vi "RealSense_HelloWorld_PointCloud Plus4.vi"() -> ()   [LabVIEW 2018]
doc: "Simple Demo showing how to connect a RealSense Camera to stream COLOR and DEPTH from the stereo camera of a D4xx series camera."
uses:
  <vilib>/Utility/miscctls.llb/LV3DPointTypeDef.ctl
  <vilib>/Utility/miscctls.llb/LVRGBAColorTypeDef.ctl
  libRealSense3.lvlib
  <vilib>/picture/3D Picture Control/NI_3D Picture Control.lvlib
panel:
  in  "Color format":enum16{"Monochrome", "RGB internal (RGB)"}(ring)
  in  "Display tab":T1(tab)
  out "depthUnits, um":i32=1000
  out "Stream selection":u16(ring)=5 items=["Depth + Left Color", "Unrectified L + R", "Rectified L + R", "Depth Only", "RGB ext. Only", "Depth + L Monochrome"]
  out "Found \nRealSense":bool=TRUE
  out "height, Y":i32=720
  out "width, X":i32=1280
  out "init results":T2={"camera name"="Intel RealSense D415", "camera S/N"="725112060262", "F/W"="05.09.11.00", "Sensor name"="Stereo Module", "api_version"=21100, "rscontext"=2785200371920, "device_list"=2783287753264, "device count"=2, "Dev out"=2783189103904, "sensor_list"=2783189110816, "sensor count"=2, "Sensor out"=2783184370480}
  in  "Select Resolution":u16(ring)=27 items=["424 x 240 @6fps", "424 x 240 @15fps", "424 x 240 @30fps", "424 x 240 @60fps", "424 x 240 @90fps", "480 x 270 @6fps", "480 x 270 @15fps", "480 x 270 @30fps", "480 x 270 @60fps", "480 x 270 @90fps", "640 x 360 @6fps", "640 x 360 @15fps", "640 x 360 @30fps", "640 x 360 @60fps", "640 x 360 @90fps", "640 x 480 @6fps", "640 x 480 @15fps", "640 x 480 @30fps", "640 x 480 @60fps", "640 x 480 @90fps", "848 x 100 @100fps", "848 x 480 @6fps", "848 x 480 @15fps", "848 x 480 @30fps", "848 x 480 @60fps", "848 x 480 @90fps", "1280 x 720 @6fps", "1280 x 720 @15fps", "1280 x 720 @30fps", "1280 x 800 @15fps", "1280 x 800 @30fps"]
  in  "Sensor index":i32
  in  "Device index":i32
  out "L-R Baseline, mm":sgl=55.142326
  out "fy":sgl=949.24713 format="%#_5g"
  out "fx":sgl=949.24713 format="%#_5g"
  out "ppy":sgl=364.42218 format="%#_5g"
  out "ppx":sgl=632.0836 format="%#_5g"
  out "Processed intrin out":T3={"width"=640, "height"=360, "ppx"=316.0418, "ppy"=182.21109, "fx"=474.62357, "fy"=474.62357, "model"=4, "coeffs[0]"=0.0, "coeffs[1]"=0.0, "coeffs[2]"=0.0, "coeffs[3]"=0.0, "coeffs[4]"=0.0} {"model" items=["RS_DISTORTION_NONE", "RS_DISTORTION_MODIFIED_BROWN_CONRADY", "RS_DISTORTION_INVERSE_BROWN_CONRADY", "RS_DISTORTION_FTHETA", "RS_DISTORTION_BROWN_CONRADY", "RS_DISTORTION_COUNT"]}
  in  "Exposure,us":sgl=33000.0
  in  "Autoexposure":bool=TRUE
  in  "Depth Presets":T4(ring)=enum."High Density"
  in  "Color Presets":T5(ring)=enum."DS410 (DS5a) 4"
  in  "Laser on/off":bool=TRUE
  in  "Gain(16-248)":sgl=16.0 min=16 max=248
  in  "Update Presets":bool
  in  "Laser \nPower (mW)":dbl(slide)=155.72448 min=0.0 max=360.0 scale=0.36..360.0
  in  "Range Scale":enum16{"200m", "100m", "60m", "6m", "2m", "1m"}(ring)=enum."6m"
  out "RGB image":picture
  out "Depth map":sgl[][](graph)
  in  "PostProcess":bool=TRUE
  out "Processing times":T6={"subsample, ms"=4, "depth-to-disp, ms"=1, "spatial filter, ms"=5, "temporal filter, ms"=1, "disp-to-depth, ms"=0}
  in  "Post-processing":T7={"Subsample"=TRUE, "Spatial filter"=TRUE, "Temporal filter"=TRUE}
  in  "Filter settings":T8={"Decimation Scale (1-10)"=3, "Spatial Alpha\n(0-1)"=0.6, "Spatial Delta \n(1/32 disp)"=8, "Temporal Alpha\n(0-1)"=0.4, "Temporal Delta\n(1/32 disp)"=20, "Persistence (0= none, 8=max)"=0, "spatial holefill radius\n(0 disable, 5 max) "=0, "spatial iteration\n(2=default)"=2} {"spatial iteration\n(2=default)" min=1 max=10; "Decimation Scale (1-10)" min=1 max=10; "Spatial Alpha\n(0-1)" min=0 max=1 format="%_2g"; "Spatial Delta \n(1/32 disp)" min=1; "Temporal Alpha\n(0-1)" min=0 max=1 format="%_2g"; "Temporal Delta\n(1/32 disp)" min=1; "Persistence (0= none, 8=max)" max=8; "spatial holefill radius\n(0 disable, 5 max)" max=6}
  out "3D Picture":refnum<vi>(3d-picture)
  in  "Texture":bool=TRUE
  out "Depth height":i32=360
  out "Depth width":i32=640
  out "Color Width":i32=1280
  out "Color Height":i32=720
  out "init error":string="No Error\rNo Error\rNo Error\rNo Error\rNo Error\rNo Error\rNo Error\rNo Error\rNo Error\rNo Error\rNo Error"
  out "Capture2 error":string="No Error"
  out "Start Error":string="No Error\rNo Error\rNo Error"
  out "Config error":string="No Error\rNo Error"
  out "Capture1 Error":string="No Error"
  out "Close Error":string="No Error\rNo Error\rNo Error\rNo Error"
  out "iteration":i32=29
  in  "stop":bool=TRUE
  # "RealSense Hello World: PointCloud & Post Processing"
  # "This demo shows how to connect a RealSense D4xx Stereo Depth Camera, and display the textured PointCloud."
  # "Note; When you change Depth Preset you need to stop and restart for the HDAD settings to take effect.\n\nTry the Color preset called \"Remove IR2\". It will remove the laser projector from the RGB 1280x720 image."
  # "INTRINSICS & EXTRINSICS"
  # "SELECT THE RESOLUTION"
  # "Recommendation:\nFor D435: 848x480, D415: 1280x720"
  # "DEPTH MAP"
  # "COLOR"
  # "Changes Color scale for Depth Map."
  # "20-1660000"
  # "3D POINTCLOUD"
  # "Rotate: Drag image\nMove X-Y: HOLD DOWN CTRL while dragging.\nZoom: SHIFT while dragging."
  # "ERRORS"
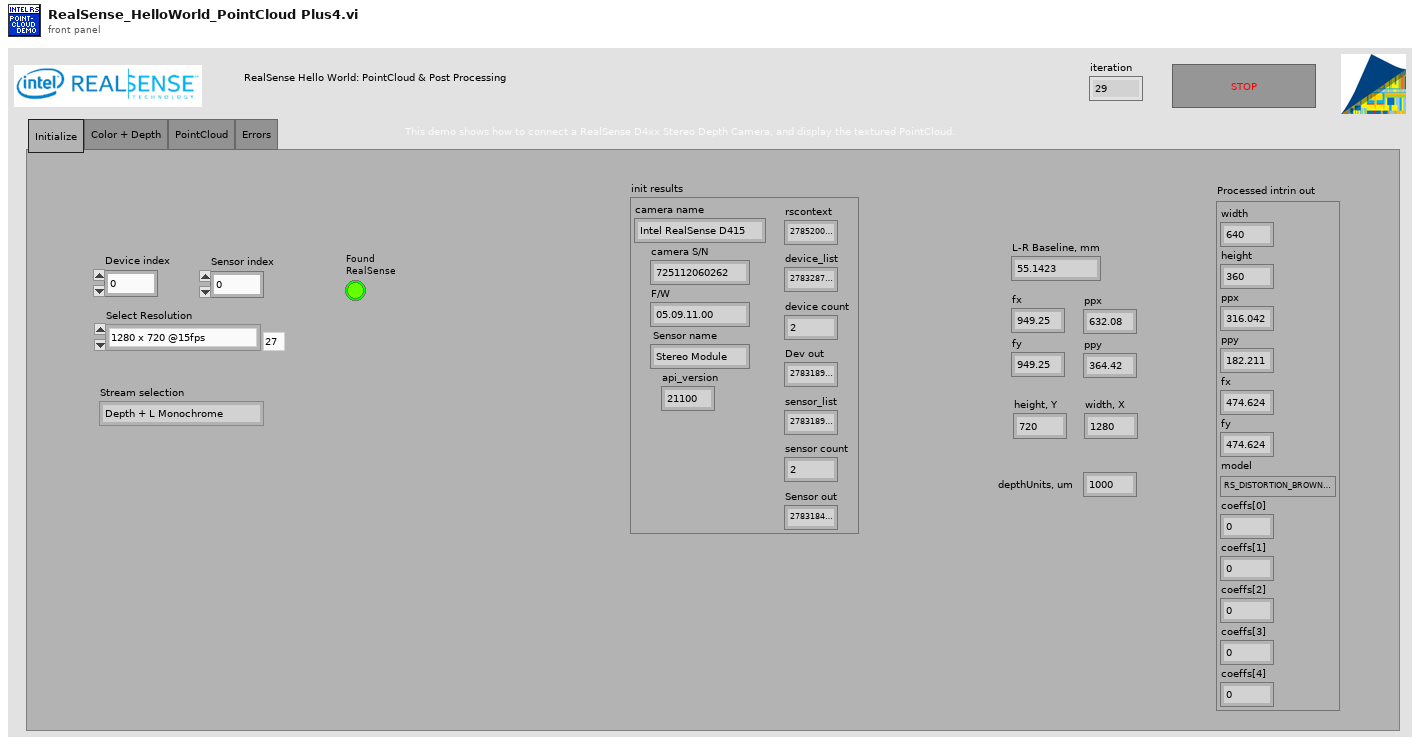
[diagram p1: front panel]
types:
  T1 = enum32{"Initialize", "Color + Depth", "PointCloud", "Errors"}
  T2 = cluster{"camera name":string, "camera S/N":string, "F/W":string, "Sensor name":string, "api_version":i32, "rscontext":u64, "device_list":u64, "device count":i32, "Dev out":u64, "sensor_list":u64, "sensor count":i32, "Sensor out":u64}
  T3 = cluster{"width":i32, "height":i32, "ppx":sgl, "ppy":sgl, "fx":sgl, "fy":sgl, "model":u32, "coeffs[0]":sgl, "coeffs[1]":sgl, "coeffs[2]":sgl, "coeffs[3]":sgl, "coeffs[4]":sgl}
  T4 = enum16{"Custom", "Original", "New Depth 1", "New Depth 2", "Depth Active 1", "Active 3D Scan", "Active Short A", "Active Short C", "Face", "Face2", "Best Box", "High Density", "Medium Density", "High Accuracy", "Hand", "Short Range", "Flat wall", "Load .JSON", "Load .JSON2"}
  T5 = enum16{"Custom", "RS400 (DS5p)", "RS400 (DS5p) 2", "RS400 (DS5p) 3", "RS400 (DS5p) 4", "RS400 (DS5p) 5", "RS410 (DS5a)", "RS410 (DS5a) 2", "DS410 (DS5a) 3", "DS410 (DS5a) 4", "DS410+IR", "DS5LR", "DS5LR-2", "DS5LR no pattern", "RS410 Remove IR", "RS410 Remove IR 2", "DS5micro", "D435"}
  T6 = cluster{"subsample, ms":u32, "depth-to-disp, ms":u32, "spatial filter, ms":u32, "temporal filter, ms":u32, "disp-to-depth, ms":u32}
  T7 = cluster{"Subsample":bool, "Spatial filter":bool, "Temporal filter":bool}
  T8 = cluster{"Decimation Scale (1-10)":u8, "Spatial Alpha\n(0-1)":sgl, "Spatial Delta \n(1/32 disp)":u16, "Temporal Alpha\n(0-1)":sgl, "Temporal Delta\n(1/32 disp)":u16, "Persistence (0= none, 8=max)":u8, "spatial holefill radius\n(0 disable, 5 max) ":u8, "spatial iteration\n(2=default)":u8}
  T9 = cluster{"Decimation Scale (1-10)":u8, "Spatial Alpha\n(0-1)":sgl, "Spatial Delta \n(1/32 disp)":u16, "Temporal Alpha\n(0-1)":sgl, "Temporal Delta\n(1/32 disp)":u16, "Persistence (0= none, 8=max)":u8, "spatial holefill radius\n(0 disable, 6 max) ":u8, "spatial iteration\n(2=default)":u8}
  T10 = cluster{"width":i32, "height":i32, "fps":i32, "Profile":u64, "ppx":sgl, "ppy":sgl, "fx":sgl, "fy":sgl, "model":u32}
  T11 = cluster{"decimation filter queue":u64, "spatial filter queue":u64, "temporal filter queue":u64, "disparity_transforg_2_queue":u64, "disparity_transforg_1_queue":u64}
  T12 = cluster{"decimation filter block":u64, "spatial filter block":u64, "temporal filter block":u64, "disparity_transforg_2_block":u64, "disparity_transforg_1_block":u64}
  T13 = enum16{"Points", "Lines", "Line Strip", "Line Loop", "Triangles", "Triangle Strip", "Triangle Fan", "Quads", "Quad Strip", "Polygon"}
  T14 = typedef "LVRGBAColorTypeDef.ctl" = cluster{"Red":sgl, "Green":sgl, "Blue":sgl, "Alpha":sgl}
  T15 = enum16{"Overall", "Per Primitive", "Per Vertex", "Binding Off"}
  T16 = cluster{"Decimation Scale (1-10)":bool, "Spatial Alpha\n(0-1)":bool, "Spatial Delta \n(1/32 disp)":bool, "Temporal Alpha\n(0-1)":bool, "Temporal Delta\n(1/32 disp)":bool, "Persistence (0= none, 8=max)":bool, bool, "spatial iteration\n(2=default)":bool}
  T17 = enum16{"Depth", "Color (ext.)", "Color (left) ", "IR Left", "IR Right", "IR Left (Y16)", "IR Right (Y16)"}
  T18 = cluster{"R":dbl, "G":dbl, "B":dbl, "Alpha":dbl}[]
  T19 = typedef "LV3DPointTypeDef.ctl" = cluster{"X":sgl, "Y":sgl, "Z":sgl}
  T20 = cluster{"Alpha":sgl, "Blue":sgl, "Green":sgl, "Red":sgl}
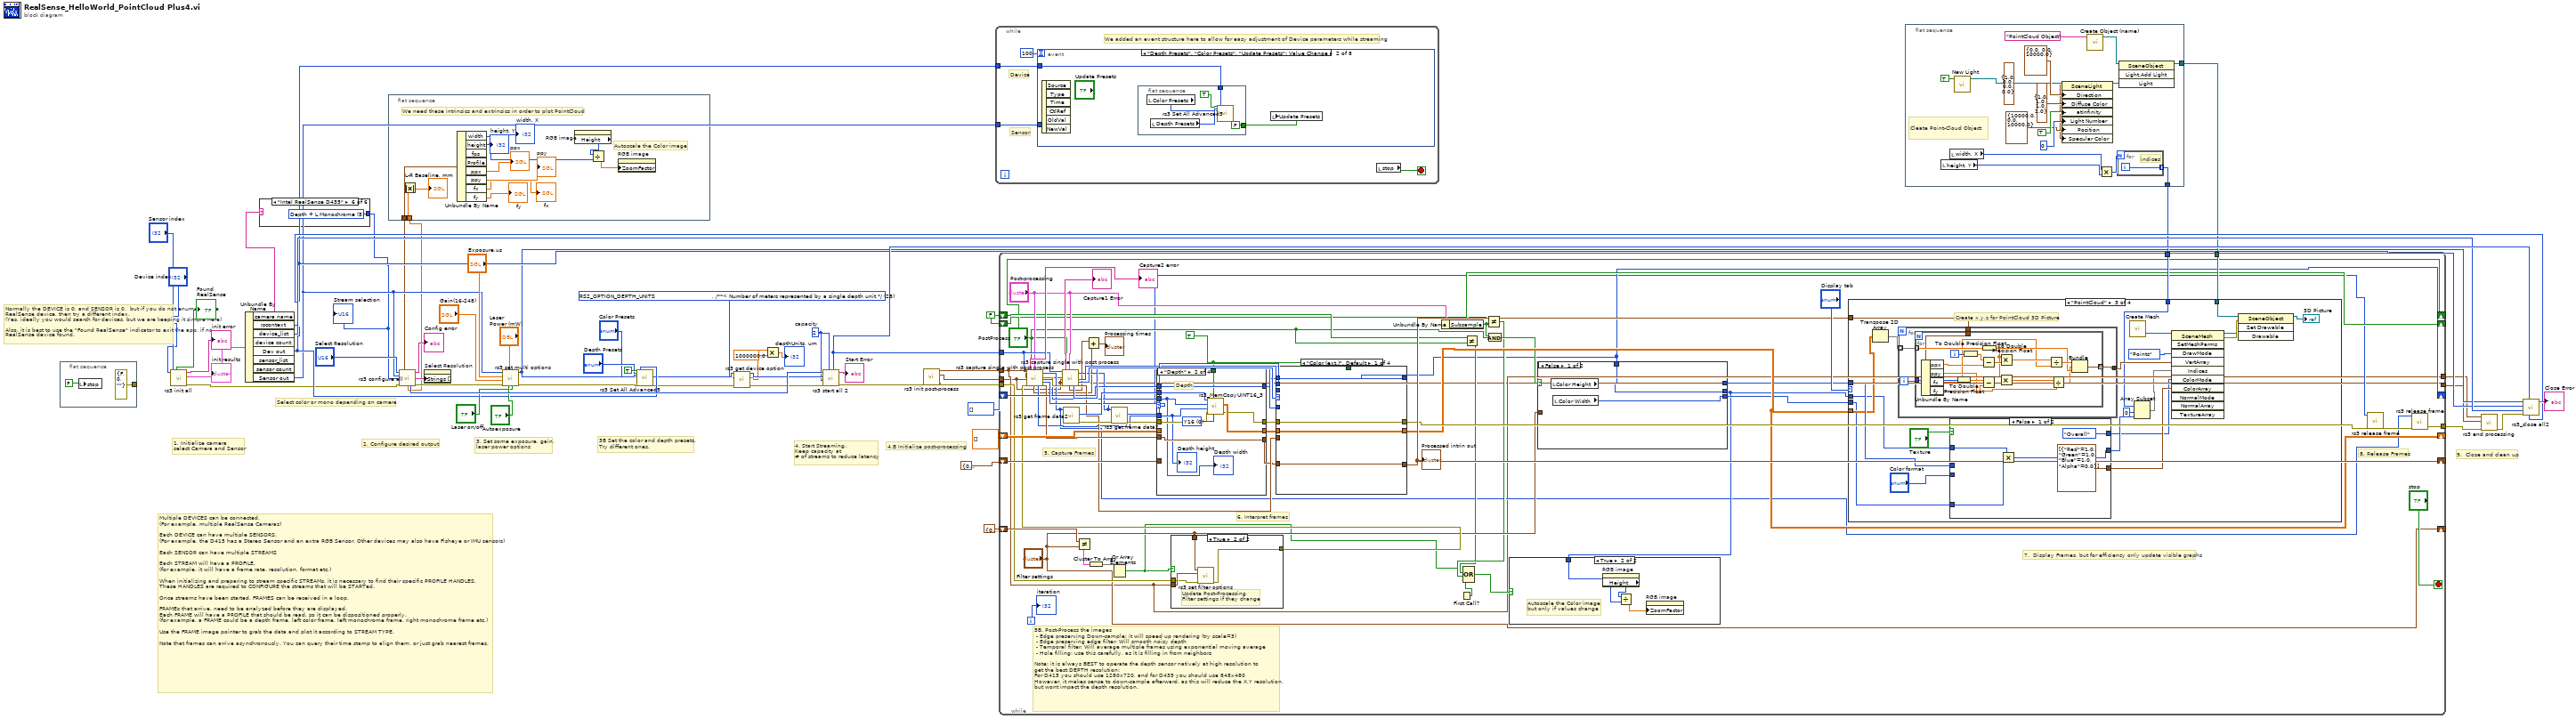
[diagram p0: block diagram]
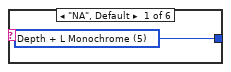
[diagram p2: hidden frame]
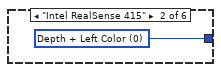
[diagram p3: hidden frame]
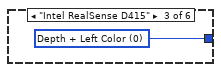
[diagram p4: hidden frame]
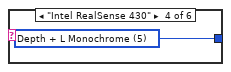
[diagram p5: hidden frame]
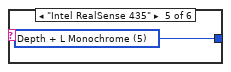
[diagram p6: hidden frame]
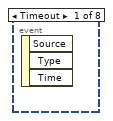
[diagram p7: hidden frame]
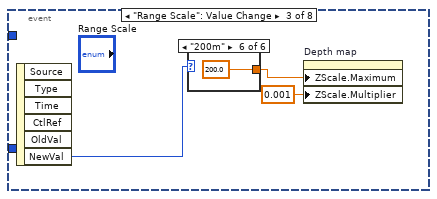
[diagram p8: hidden frame]
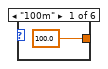
[diagram p9: hidden frame]
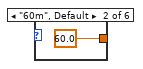
[diagram p10: hidden frame]
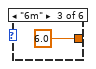
[diagram p11: hidden frame]
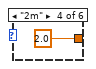
[diagram p12: hidden frame]
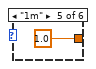
[diagram p13: hidden frame]
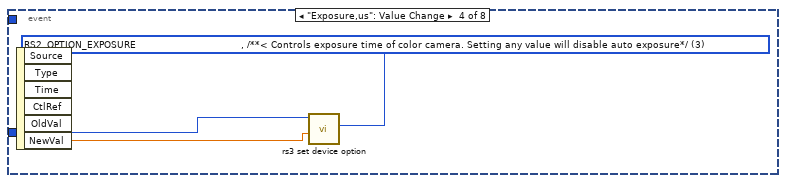
[diagram p14: hidden frame]
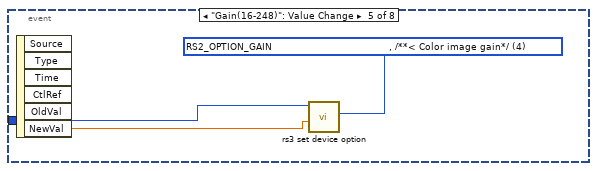
[diagram p15: hidden frame]
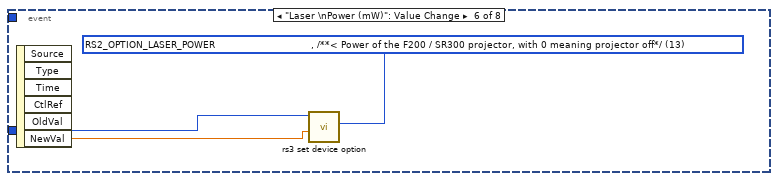
[diagram p16: hidden frame]
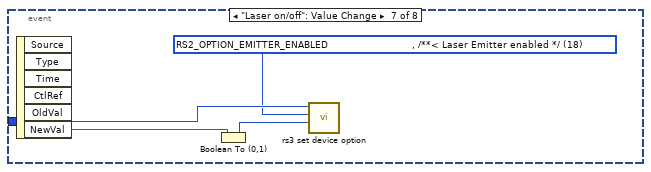
[diagram p17: hidden frame]
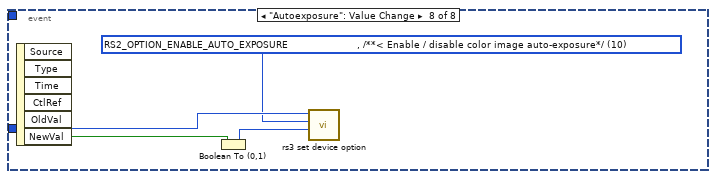
[diagram p18: hidden frame]
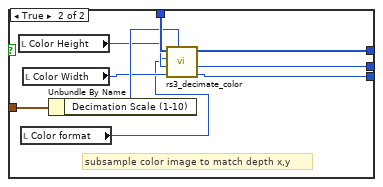
[diagram p20: hidden frame]
diagram:
  w6 = FALSE ("PostProcess")
  w13 = 2  # capacity
  w17 = u16 28 items=["    RS2_OPTION_BACKLIGHT_COMPENSATION                     , /**< Enable / disable color backlight compensation*/", "    RS2_OPTION_BRIGHTNESS                                 , /**< Color image brightness*/", "    RS2_OPTION_CONTRAST                                   , /**< Color image contrast*/", "    RS2_OPTION_EXPOSURE                                   , /**< Controls exposure time of color camera. Setting any value will disable auto exposure*/", "    RS2_OPTION_GAIN                                       , /**< Color image gain*/", "    RS2_OPTION_GAMMA                                      , /**< Color image gamma setting*/", "    RS2_OPTION_HUE                                        , /**< Color image hue*/", "    RS2_OPTION_SATURATION                                 , /**< Color image saturation setting*/", "    RS2_OPTION_SHARPNESS                                  , /**< Color image sharpness setting*/", "    RS2_OPTION_WHITE_BALANCE                              , /**< Controls white balance of color image. Setting any value will disable auto white balance*/", "    RS2_OPTION_ENABLE_AUTO_EXPOSURE                       , /**< Enable / disable color image auto-exposure*/", "    RS2_OPTION_ENABLE_AUTO_WHITE_BALANCE                  , /**< Enable / disable color image auto-white-balance*/", "    RS2_OPTION_VISUAL_PRESET                              , /**< Provide access to several recommend sets of option presets for the depth camera */", "    RS2_OPTION_LASER_POWER                                , /**< Power of the F200 / SR300 projector, with 0 meaning projector off*/", "    RS2_OPTION_ACCURACY                                   , /**< Set the number of patterns projected per frame. The higher the accuracy value the more patterns projected. Increasing the number of patterns help to achieve better accuracy. Note that this c", "    RS2_OPTION_MOTION_RANGE                               , /**< Motion vs. Range trade-off, with lower values allowing for better motion sensitivity and higher values allowing for better depth range*/", "    RS2_OPTION_FILTER_OPTION                              , /**< Set the filter to apply to each depth frame. Each one of the filter is optimized per the application requirements*/", "    RS2_OPTION_CONFIDENCE_THRESHOLD                       , /**< The confidence level threshold used by the Depth algorithm pipe to set whether a pixel will get a valid range or will be marked with invalid range*/", "    RS2_OPTION_EMITTER_ENABLED                            , /**< Laser Emitter enabled */", "    RS2_OPTION_FRAMES_QUEUE_SIZE                          , /**< Number of frames the user is allowed to keep per stream. Trying to hold-on to more frames will cause frame-drops.*/", "    RS2_OPTION_TOTAL_FRAME_DROPS                          , /**< Total number of detected frame drops from all streams */", "    RS2_OPTION_AUTO_EXPOSURE_MODE                         , /**< Auto-Exposure modes: Static, Anti-Flicker and Hybrid */", "    RS2_OPTION_POWER_LINE_FREQUENCY                       , /**< Power Line Frequency control for anti-flickering Off/50Hz/60Hz/Auto */", "    RS2_OPTION_ASIC_TEMPERATURE                           , /**< Current Asic Temperature */", "    RS2_OPTION_ERROR_POLLING_ENABLED                      , /**< disable error handling */", "    RS2_OPTION_PROJECTOR_TEMPERATURE                      , /**< Current Projector Temperature */", "    RS2_OPTION_OUTPUT_TRIGGER_ENABLED                     , /**< Enable / disable trigger to be outputed from the camera to any external device on every depth frame */", "    RS2_OPTION_MOTION_MODULE_TEMPERATURE                  , /**< Current Motion-Module Temperature */", "    RS2_OPTION_DEPTH_UNITS                                , /**< Number of meters represented by a single depth unit */", "    RS2_OPTION_ENABLE_MOTION_CORRECTION                   , /**< Enable/Disable automatic correction of the motion data */", "    RS2_OPTION_AUTO_EXPOSURE_PRIORITY                     , /**< Allows sensor to dynamically ajust the frame rate depending on lighting conditions */", "    RS2_OPTION_COLOR_SCHEME                               , /**< Color scheme for data visualization */", "    RS2_OPTION_HISTOGRAM_EQUALIZATION_ENABLED             , /**< Perform histogram equalization post-processing on the depth data */", "    RS2_OPTION_MIN_DISTANCE                               , /**< Minimal distance to the target */", "    RS2_OPTION_MAX_DISTANCE                               , /**< Maximum distance to the target */", "    RS2_OPTION_TEXTURE_SOURCE                             , /**< Texture mapping stream unique ID */", "    RS2_OPTION_FILTER_MAGNITUDE                           , /**< The 2D-filter effect. The specific interpretation is given within the context of the filter */", "    RS2_OPTION_FILTER_SMOOTH_ALPHA                        , /**< 2D-filter parameter controls the weight/radius for smoothing.*/", "    RS2_OPTION_FILTER_SMOOTH_DELTA                        , /**< 2D-filter range/validity threshold*/", "    RS2_OPTION_HOLES_FILL                                 , /**< Enhance depth data post-processing with holes filling where appropriate*/", "    RS2_OPTION_STEREO_BASELINE                            , /**< The distance in mm between the first and the second imagers in stereo-based depth cameras*/", "    RS2_OPTION_AUTO_EXPOSURE_CONVERGE_STEP                , /**< Allows dynamically ajust the converge step value of the target exposure in Auto-Exposure algorithm*/", "    RS2_OPTION_COUNT                                        /**< Number of enumeration values. Not a valid input: intended to be used in for-loops. */"] ("RS Option")
  # "4.B Initialize post-processing"
  # "4. Start Streaming. \nKeep capacity at \n# of streams to reduce latency"
  # "3B Set the color and depth presets.\nTry different ones."
  # "Select color or mono depending on camera"
  # "Normally the DEVICE is 0, and SENSOR is 0,  but if you do not enumerate the RealSense device, then try a different index.\n(Yes, ideally you would search for devices, but we are keeping it simple here)\n\nAlso, it is best to use the \"Found RealSense\" indicator to exit the app, if no RealSense device found."
  # "Multiple DEVICES can be connected. \n(For example, multiple RealSense Cameras)\n\nEach DEVICE can have multiple SENSORS. \n(For example, the D415 has a Stereo Sensor and an extra RGB Sensor. Other devices may also have Fisheye or IMU sensors) \n\nEach SENSOR can have multiple STREAMS\n\nEach STREAM will have a PROFILE. \n(for example, it will have a frame rate, resolution, format etc.)\n\nWhen initializing and preparing to stream specific STREAMs, it is necessary to find their specific PROFILE HANDLES.\nThese HANDLES are required to CONFIGURE the streams that will be STARTed. \n\nOnce streams have been started, FRAMES can be received in a loop. \n \nFRAMEs that arrive, need to be analyzed before they are displayed. \nEach FRAME will have a PROFILE that should be read, so it can be dispositioned properly.\n(for example, a FRAME could be a depth frame, left color frame, left monochrome frame, right monochrome frame etc.)\n\nUse the FRAME image pointer to grab the data and plot it according to STREAM TYPE.\n\nNote that frames can arrive asynchronously. You can query their time stamp to align them, or just grab nearest frames."
  # "9.  Close and clean up"
  # "3. Set some exposure, gain, \nlaser power options"
  # "2. Configure desired output"
  # "1. Initialize camera\nselect Camera and Sensor"
  n1 = flat-sequence {
    tunnel: [errorcluster {"status"=FALSE, "code"=0, "source"=""} ("error in")] -> _
    frame #0 {
      n2 = local write "stop"(FALSE ("stop")) -> ()
    }
  }
  n3 = call "rs3 init all.vi"("Select Device"="Device index", "Select Sensor"="Sensor index") -> ("error out"=w23:errorcluster, "init results"=w28:T2, "init error"=→"init error":string, "Found RealSense"=→"Found \nRealSense":bool)  [unwired: 3 in, 3 out]
  "init results" <- w28
  n4 = Unbundle By Name(w28) -> ("camera name"=w22:string, "rscontext"=w50:u64, "device_list"=w51:u64, "Dev out"=w36:u64, "Sensor out"=w35:u64)  [unwired: 3 out]
  n5 = case shown="\"Intel RealSense D435\"" w22 {
    tunnel: [w58 w59 w60 w61 w62 w63] -> w5
    frame "NA", Default {
      w58 = u16 5 items=["Depth + Left Color", "Unrectified L + R", "Rectified L + R", "Depth Only", "RGB ext. Only", "Depth + L Monochrome"] ("Stream selection")
    }
    frame "Intel RealSense 415" {
      w59 = u16 0 items=["Depth + Left Color", "Unrectified L + R", "Rectified L + R", "Depth Only", "RGB ext. Only", "Depth + L Monochrome"] ("Stream selection")
    }
    frame "Intel RealSense D415" {
      w60 = u16 0 items=["Depth + Left Color", "Unrectified L + R", "Rectified L + R", "Depth Only", "RGB ext. Only", "Depth + L Monochrome"] ("Stream selection")
    }
    frame "Intel RealSense 430" {
      w61 = u16 5 items=["Depth + Left Color", "Unrectified L + R", "Rectified L + R", "Depth Only", "RGB ext. Only", "Depth + L Monochrome"] ("Stream selection")
    }
    frame "Intel RealSense 435" {
      w62 = u16 5 items=["Depth + Left Color", "Unrectified L + R", "Rectified L + R", "Depth Only", "RGB ext. Only", "Depth + L Monochrome"] ("Stream selection")
    }
    frame "Intel RealSense D435" {
      w63 = u16 5 items=["Depth + Left Color", "Unrectified L + R", "Rectified L + R", "Depth Only", "RGB ext. Only", "Depth + L Monochrome"] ("Stream selection")
    }
  }
  "Stream selection" <- w5
  n6 = flat-sequence {
    tunnel: w33 -> [w74]
    tunnel: w32 -> [w73]
    frame #0 {
      # "Autoscale the Color image"
      # "We need these intrinsics and extrinsics in order to plot PointCloud"
      n7 = Absolute Value(x=w74) -> (abs(x)=→"L-R Baseline, mm":sgl)
      n8 = Unbundle By Name(w73) -> ("width"=→"width, X":i32, "height"=w71:i32, "ppx"=→"ppx":sgl, "ppy"=→"ppy":sgl, "fx"=→"fx":sgl, "fy"=→"fy":sgl)  [unwired: 2 out]
      "height, Y" <- w71
      n9 = property on="RGB image" class="Pict"() -> ("Height"=w72:u32)  [unwired: 2 in, 2 out]
      n10 = Divide(x=w72, y=w71) -> (x/y=w70:dbl)
      n11 = property on="RGB image" class="Pict"("ZoomFactor"=w70) -> ()  [unwired: 2 in, 2 out]
    }
  }
  n12 = call "rs3 configure all.vi"("Select Resolution"="Select Resolution", "Sensor in"=w35, "Stream selection"=w5, "error in (no error)"=w23) -> ("Output stream L"=w32:T10, "config error"=→"Config error":string, "Output stream"=w47:string[], "L-R Baseline, mm"=w33:sgl, "Stream Profile Handles"=w55:u64[], "error out"=w46:errorcluster)  [unwired: 2 in, 4 out]
  n13 = property on="Select Resolution" class="Ring (strict)"("Strings []"=w47) -> ()  [unwired: 2 in, 2 out]
  n14 = call "rs3 set multi options.vi"("laser on/off"="Laser on/off", "autoexposure"="Autoexposure", "Laser power, mW (0-360)"="Laser \nPower (mW)", "error in (no error)"=w46, "Gain(16-248)"="Gain(16-248)", "Exposure, us"="Exposure,us", "Sensor in"=w35) -> ("error out"=w40:errorcluster, "Sensor out"=w19:u64)  [unwired: 2 in, 1 out]
  n15 = call "rs3 Set All Advanced5.vi"("Set Color Corr"=TRUE, "Depth Presets"="Depth Presets", "Color Presets"="Color Presets", "error in (no error)"=w40, "device in"=w36) -> ("error out"=w21:errorcluster)  [unwired: 20 in, 2 out]
  n16 = call "rs3 get device option.vi"("error in (no error)"=w21, "RS Option"=w17, "sensor in"=w19) -> ("error out"=w20:errorcluster, "option return"=w16:dbl, "sensor out"=w18:u64)  [unwired: 4 in, 2 out]
  n17 = Multiply(x=w16, y=1000000.0) -> (x*y=→"depthUnits, um":dbl)
  n18 = call "rs3 start all 2.vi"("capacity"=w13, "error in (no error)"=w20, "Count of Streams"=w13, "Sensor in"=w18, "Stream profile array"=w55) -> ("error out"=w12:errorcluster, "Config Error"=→"Start Error":string, "queue out"=w54:u64)  [unwired: 3 in, 1 out]
  n19 = call "rs3 init post-process.vi"("error in (no error)"=w12) -> ("error out"=w7:errorcluster, "Processing Queues"=w11:T11, "Processing Blocks"=w10:T12)  [unwired: 8 in]
  n20 = while {
    tunnel: w36 -> [w77]
    tunnel: w35 -> [w76]
    stop <- w78 stop-if-true
    # "Sensor"
    # "Device"
    # "We added an event structure here to allow for easy adjustment of Device parameters while streaming"
    n21 = event shown="[1] \"Depth Presets\", \"Color Presets\", \"Update Presets\": Value Change" {
      selector: _ -> [_ _ _ _ _ _ _ _]
      dyn-events: _ -> [_ _ _ _ _ _ _ _]
      timeout: 100 -> [_ _ _ _ _ _ _ _]
      tunnel: w77 -> [_ w80 _ _ _ _ _ _]
      tunnel: w76 -> [_ _ _ w97 w100 w103 w107 w111]
      event Timeout {
        n22 = event-data() -> ()  [unwired: 1 in, 3 out]
      }
      event "Depth Presets", "Color Presets", "Update Presets": Value Change {
        n23 = event-data() -> ()  [unwired: 1 in, 6 out]
        n24 = flat-sequence {
          tunnel: w80 -> [w82]
          tunnel: [FALSE ("Update Presets")] -> w79
          frame #0 {
            n25 = local read "Color Presets"() -> (w84:T5)
            n26 = local read "Depth Presets"() -> (w85:T4)
            n27 = call "rs3 Set All Advanced5.vi"("Set Color Corr"=TRUE, "Depth Presets"=w85, "Color Presets"=w84, "device in"=w82) -> ()  [unwired: 21 in, 3 out]
          }
        }
        n28 = local write "Update Presets"(w79) -> ()
      }
      event "Range Scale": Value Change {
        n29 = event-data() -> ("NewVal"=w87:enum16{"200m", "100m", "60m", "6m", "2m", "1m"})  [unwired: 1 in, 5 out]
        n30 = case shown="\"200m\"" w87 {
          tunnel: [100.0 ("Z Scale.Offset and Multiplier:Multiplier") 60.0 ("Z Scale.Offset and Multiplier:Multiplier") 6.0 ("Z Scale.Offset and Multiplier:Multiplier") 2.0 ("Z Scale.Offset and Multiplier:Multiplier") 1.0 ("Z Scale.Offset and Multiplier:Multiplier") 200.0 ("Z Scale.Offset and Multiplier:Multiplier")] -> w86
          frame "100m" {
          }
          frame "60m", Default {
          }
          frame "6m" {
          }
          frame "2m" {
          }
          frame "1m" {
          }
          frame "200m" {
          }
        }
        n31 = property on="Depth map" class="IntGraph (strict)"("ZScale.Maximum"=w86, "ZScale.Multiplier"=0.001 ("Z Scale.Offset and Multiplier:Multiplier")) -> ()  [unwired: 2 in, 2 out]
      }
      event "Exposure,us": Value Change {
        w95 = u16 3 items=["    RS2_OPTION_BACKLIGHT_COMPENSATION                     , /**< Enable / disable color backlight compensation*/", "    RS2_OPTION_BRIGHTNESS                                 , /**< Color image brightness*/", "    RS2_OPTION_CONTRAST                                   , /**< Color image contrast*/", "    RS2_OPTION_EXPOSURE                                   , /**< Controls exposure time of color camera. Setting any value will disable auto exposure*/", "    RS2_OPTION_GAIN                                       , /**< Color image gain*/", "    RS2_OPTION_GAMMA                                      , /**< Color image gamma setting*/", "    RS2_OPTION_HUE                                        , /**< Color image hue*/", "    RS2_OPTION_SATURATION                                 , /**< Color image saturation setting*/", "    RS2_OPTION_SHARPNESS                                  , /**< Color image sharpness setting*/", "    RS2_OPTION_WHITE_BALANCE                              , /**< Controls white balance of color image. Setting any value will disable auto white balance*/", "    RS2_OPTION_ENABLE_AUTO_EXPOSURE                       , /**< Enable / disable color image auto-exposure*/", "    RS2_OPTION_ENABLE_AUTO_WHITE_BALANCE                  , /**< Enable / disable color image auto-white-balance*/", "    RS2_OPTION_VISUAL_PRESET                              , /**< Provide access to several recommend sets of option presets for the depth camera */", "    RS2_OPTION_LASER_POWER                                , /**< Power of the F200 / SR300 projector, with 0 meaning projector off*/", "    RS2_OPTION_ACCURACY                                   , /**< Set the number of patterns projected per frame. The higher the accuracy value the more patterns projected. Increasing the number of patterns help to achieve better accuracy. Note that this c", "    RS2_OPTION_MOTION_RANGE                               , /**< Motion vs. Range trade-off, with lower values allowing for better motion sensitivity and higher values allowing for better depth range*/", "    RS2_OPTION_FILTER_OPTION                              , /**< Set the filter to apply to each depth frame. Each one of the filter is optimized per the application requirements*/", "    RS2_OPTION_CONFIDENCE_THRESHOLD                       , /**< The confidence level threshold used by the Depth algorithm pipe to set whether a pixel will get a valid range or will be marked with invalid range*/", "    RS2_OPTION_EMITTER_ENABLED                            , /**< Laser Emitter enabled */", "    RS2_OPTION_FRAMES_QUEUE_SIZE                          , /**< Number of frames the user is allowed to keep per stream. Trying to hold-on to more frames will cause frame-drops.*/", "    RS2_OPTION_TOTAL_FRAME_DROPS                          , /**< Total number of detected frame drops from all streams */", "    RS2_OPTION_AUTO_EXPOSURE_MODE                         , /**< Auto-Exposure modes: Static, Anti-Flicker and Hybrid */", "    RS2_OPTION_POWER_LINE_FREQUENCY                       , /**< Power Line Frequency control for anti-flickering Off/50Hz/60Hz/Auto */", "    RS2_OPTION_ASIC_TEMPERATURE                           , /**< Current Asic Temperature */", "    RS2_OPTION_ERROR_POLLING_ENABLED                      , /**< disable error handling */", "    RS2_OPTION_PROJECTOR_TEMPERATURE                      , /**< Current Projector Temperature */", "    RS2_OPTION_OUTPUT_TRIGGER_ENABLED                     , /**< Enable / disable trigger to be outputed from the camera to any external device on every depth frame */", "    RS2_OPTION_MOTION_MODULE_TEMPERATURE                  , /**< Current Motion-Module Temperature */", "    RS2_OPTION_DEPTH_UNITS                                , /**< Number of meters represented by a single depth unit */", "    RS2_OPTION_ENABLE_MOTION_CORRECTION                   , /**< Enable/Disable automatic correction of the motion data */", "    RS2_OPTION_AUTO_EXPOSURE_PRIORITY                     , /**< Allows sensor to dynamically ajust the frame rate depending on lighting conditions */", "    RS2_OPTION_COUNT                                      , /**< Number of enumeration values. Not a valid input: intended to be used in for-loops. */"] ("RS Option")
        n32 = event-data() -> ("NewVal"=w96:sgl)  [unwired: 1 in, 5 out]
        n33 = call "rs3 set device option.vi"("value"=w96, "RS Option"=w95, "Sensor in"=w97) -> ()  [unwired: 6 in, 3 out]
      }
      event "Gain(16-248)": Value Change {
        w98 = u16 4 items=["    RS2_OPTION_BACKLIGHT_COMPENSATION                     , /**< Enable / disable color backlight compensation*/", "    RS2_OPTION_BRIGHTNESS                                 , /**< Color image brightness*/", "    RS2_OPTION_CONTRAST                                   , /**< Color image contrast*/", "    RS2_OPTION_EXPOSURE                                   , /**< Controls exposure time of color camera. Setting any value will disable auto exposure*/", "    RS2_OPTION_GAIN                                       , /**< Color image gain*/", "    RS2_OPTION_GAMMA                                      , /**< Color image gamma setting*/", "    RS2_OPTION_HUE                                        , /**< Color image hue*/", "    RS2_OPTION_SATURATION                                 , /**< Color image saturation setting*/", "    RS2_OPTION_SHARPNESS                                  , /**< Color image sharpness setting*/", "    RS2_OPTION_WHITE_BALANCE                              , /**< Controls white balance of color image. Setting any value will disable auto white balance*/", "    RS2_OPTION_ENABLE_AUTO_EXPOSURE                       , /**< Enable / disable color image auto-exposure*/", "    RS2_OPTION_ENABLE_AUTO_WHITE_BALANCE                  , /**< Enable / disable color image auto-white-balance*/", "    RS2_OPTION_VISUAL_PRESET                              , /**< Provide access to several recommend sets of option presets for the depth camera */", "    RS2_OPTION_LASER_POWER                                , /**< Power of the F200 / SR300 projector, with 0 meaning projector off*/", "    RS2_OPTION_ACCURACY                                   , /**< Set the number of patterns projected per frame. The higher the accuracy value the more patterns projected. Increasing the number of patterns help to achieve better accuracy. Note that this c", "    RS2_OPTION_MOTION_RANGE                               , /**< Motion vs. Range trade-off, with lower values allowing for better motion sensitivity and higher values allowing for better depth range*/", "    RS2_OPTION_FILTER_OPTION                              , /**< Set the filter to apply to each depth frame. Each one of the filter is optimized per the application requirements*/", "    RS2_OPTION_CONFIDENCE_THRESHOLD                       , /**< The confidence level threshold used by the Depth algorithm pipe to set whether a pixel will get a valid range or will be marked with invalid range*/", "    RS2_OPTION_EMITTER_ENABLED                            , /**< Laser Emitter enabled */", "    RS2_OPTION_FRAMES_QUEUE_SIZE                          , /**< Number of frames the user is allowed to keep per stream. Trying to hold-on to more frames will cause frame-drops.*/", "    RS2_OPTION_TOTAL_FRAME_DROPS                          , /**< Total number of detected frame drops from all streams */", "    RS2_OPTION_AUTO_EXPOSURE_MODE                         , /**< Auto-Exposure modes: Static, Anti-Flicker and Hybrid */", "    RS2_OPTION_POWER_LINE_FREQUENCY                       , /**< Power Line Frequency control for anti-flickering Off/50Hz/60Hz/Auto */", "    RS2_OPTION_ASIC_TEMPERATURE                           , /**< Current Asic Temperature */", "    RS2_OPTION_ERROR_POLLING_ENABLED                      , /**< disable error handling */", "    RS2_OPTION_PROJECTOR_TEMPERATURE                      , /**< Current Projector Temperature */", "    RS2_OPTION_OUTPUT_TRIGGER_ENABLED                     , /**< Enable / disable trigger to be outputed from the camera to any external device on every depth frame */", "    RS2_OPTION_MOTION_MODULE_TEMPERATURE                  , /**< Current Motion-Module Temperature */", "    RS2_OPTION_DEPTH_UNITS                                , /**< Number of meters represented by a single depth unit */", "    RS2_OPTION_ENABLE_MOTION_CORRECTION                   , /**< Enable/Disable automatic correction of the motion data */", "    RS2_OPTION_AUTO_EXPOSURE_PRIORITY                     , /**< Allows sensor to dynamically ajust the frame rate depending on lighting conditions */", "    RS2_OPTION_COUNT                                      , /**< Number of enumeration values. Not a valid input: intended to be used in for-loops. */"] ("RS Option")
        n34 = event-data() -> ("NewVal"=w99:sgl)  [unwired: 1 in, 5 out]
        n35 = call "rs3 set device option.vi"("value"=w99, "RS Option"=w98, "Sensor in"=w100) -> ()  [unwired: 6 in, 3 out]
      }
      event "Laser \nPower (mW)": Value Change {
        w101 = u16 13 items=["    RS2_OPTION_BACKLIGHT_COMPENSATION                     , /**< Enable / disable color backlight compensation*/", "    RS2_OPTION_BRIGHTNESS                                 , /**< Color image brightness*/", "    RS2_OPTION_CONTRAST                                   , /**< Color image contrast*/", "    RS2_OPTION_EXPOSURE                                   , /**< Controls exposure time of color camera. Setting any value will disable auto exposure*/", "    RS2_OPTION_GAIN                                       , /**< Color image gain*/", "    RS2_OPTION_GAMMA                                      , /**< Color image gamma setting*/", "    RS2_OPTION_HUE                                        , /**< Color image hue*/", "    RS2_OPTION_SATURATION                                 , /**< Color image saturation setting*/", "    RS2_OPTION_SHARPNESS                                  , /**< Color image sharpness setting*/", "    RS2_OPTION_WHITE_BALANCE                              , /**< Controls white balance of color image. Setting any value will disable auto white balance*/", "    RS2_OPTION_ENABLE_AUTO_EXPOSURE                       , /**< Enable / disable color image auto-exposure*/", "    RS2_OPTION_ENABLE_AUTO_WHITE_BALANCE                  , /**< Enable / disable color image auto-white-balance*/", "    RS2_OPTION_VISUAL_PRESET                              , /**< Provide access to several recommend sets of option presets for the depth camera */", "    RS2_OPTION_LASER_POWER                                , /**< Power of the F200 / SR300 projector, with 0 meaning projector off*/", "    RS2_OPTION_ACCURACY                                   , /**< Set the number of patterns projected per frame. The higher the accuracy value the more patterns projected. Increasing the number of patterns help to achieve better accuracy. Note that this c", "    RS2_OPTION_MOTION_RANGE                               , /**< Motion vs. Range trade-off, with lower values allowing for better motion sensitivity and higher values allowing for better depth range*/", "    RS2_OPTION_FILTER_OPTION                              , /**< Set the filter to apply to each depth frame. Each one of the filter is optimized per the application requirements*/", "    RS2_OPTION_CONFIDENCE_THRESHOLD                       , /**< The confidence level threshold used by the Depth algorithm pipe to set whether a pixel will get a valid range or will be marked with invalid range*/", "    RS2_OPTION_EMITTER_ENABLED                            , /**< Laser Emitter enabled */", "    RS2_OPTION_FRAMES_QUEUE_SIZE                          , /**< Number of frames the user is allowed to keep per stream. Trying to hold-on to more frames will cause frame-drops.*/", "    RS2_OPTION_TOTAL_FRAME_DROPS                          , /**< Total number of detected frame drops from all streams */", "    RS2_OPTION_AUTO_EXPOSURE_MODE                         , /**< Auto-Exposure modes: Static, Anti-Flicker and Hybrid */", "    RS2_OPTION_POWER_LINE_FREQUENCY                       , /**< Power Line Frequency control for anti-flickering Off/50Hz/60Hz/Auto */", "    RS2_OPTION_ASIC_TEMPERATURE                           , /**< Current Asic Temperature */", "    RS2_OPTION_ERROR_POLLING_ENABLED                      , /**< disable error handling */", "    RS2_OPTION_PROJECTOR_TEMPERATURE                      , /**< Current Projector Temperature */", "    RS2_OPTION_OUTPUT_TRIGGER_ENABLED                     , /**< Enable / disable trigger to be outputed from the camera to any external device on every depth frame */", "    RS2_OPTION_MOTION_MODULE_TEMPERATURE                  , /**< Current Motion-Module Temperature */", "    RS2_OPTION_DEPTH_UNITS                                , /**< Number of meters represented by a single depth unit */", "    RS2_OPTION_ENABLE_MOTION_CORRECTION                   , /**< Enable/Disable automatic correction of the motion data */", "    RS2_OPTION_AUTO_EXPOSURE_PRIORITY                     , /**< Allows sensor to dynamically ajust the frame rate depending on lighting conditions */", "    RS2_OPTION_COUNT                                      , /**< Number of enumeration values. Not a valid input: intended to be used in for-loops. */"] ("RS Option")
        n36 = event-data() -> ("NewVal"=w102:dbl)  [unwired: 1 in, 5 out]
        n37 = call "rs3 set device option.vi"("value"=w102, "RS Option"=w101, "Sensor in"=w103) -> ()  [unwired: 6 in, 3 out]
      }
      event "Laser on/off": Value Change {
        w106 = u16 18 items=["    RS2_OPTION_BACKLIGHT_COMPENSATION                     , /**< Enable / disable color backlight compensation*/", "    RS2_OPTION_BRIGHTNESS                                 , /**< Color image brightness*/", "    RS2_OPTION_CONTRAST                                   , /**< Color image contrast*/", "    RS2_OPTION_EXPOSURE                                   , /**< Controls exposure time of color camera. Setting any value will disable auto exposure*/", "    RS2_OPTION_GAIN                                       , /**< Color image gain*/", "    RS2_OPTION_GAMMA                                      , /**< Color image gamma setting*/", "    RS2_OPTION_HUE                                        , /**< Color image hue*/", "    RS2_OPTION_SATURATION                                 , /**< Color image saturation setting*/", "    RS2_OPTION_SHARPNESS                                  , /**< Color image sharpness setting*/", "    RS2_OPTION_WHITE_BALANCE                              , /**< Controls white balance of color image. Setting any value will disable auto white balance*/", "    RS2_OPTION_ENABLE_AUTO_EXPOSURE                       , /**< Enable / disable color image auto-exposure*/", "    RS2_OPTION_ENABLE_AUTO_WHITE_BALANCE                  , /**< Enable / disable color image auto-white-balance*/", "    RS2_OPTION_VISUAL_PRESET                              , /**< Provide access to several recommend sets of option presets for the depth camera */", "    RS2_OPTION_LASER_POWER                                , /**< Power of the F200 / SR300 projector, with 0 meaning projector off*/", "    RS2_OPTION_ACCURACY                                   , /**< Set the number of patterns projected per frame. The higher the accuracy value the more patterns projected. Increasing the number of patterns help to achieve better accuracy. Note that this c", "    RS2_OPTION_MOTION_RANGE                               , /**< Motion vs. Range trade-off, with lower values allowing for better motion sensitivity and higher values allowing for better depth range*/", "    RS2_OPTION_FILTER_OPTION                              , /**< Set the filter to apply to each depth frame. Each one of the filter is optimized per the application requirements*/", "    RS2_OPTION_CONFIDENCE_THRESHOLD                       , /**< The confidence level threshold used by the Depth algorithm pipe to set whether a pixel will get a valid range or will be marked with invalid range*/", "    RS2_OPTION_EMITTER_ENABLED                            , /**< Laser Emitter enabled */", "    RS2_OPTION_FRAMES_QUEUE_SIZE                          , /**< Number of frames the user is allowed to keep per stream. Trying to hold-on to more frames will cause frame-drops.*/", "    RS2_OPTION_TOTAL_FRAME_DROPS                          , /**< Total number of detected frame drops from all streams */", "    RS2_OPTION_AUTO_EXPOSURE_MODE                         , /**< Auto-Exposure modes: Static, Anti-Flicker and Hybrid */", "    RS2_OPTION_POWER_LINE_FREQUENCY                       , /**< Power Line Frequency control for anti-flickering Off/50Hz/60Hz/Auto */", "    RS2_OPTION_ASIC_TEMPERATURE                           , /**< Current Asic Temperature */", "    RS2_OPTION_ERROR_POLLING_ENABLED                      , /**< disable error handling */", "    RS2_OPTION_PROJECTOR_TEMPERATURE                      , /**< Current Projector Temperature */", "    RS2_OPTION_OUTPUT_TRIGGER_ENABLED                     , /**< Enable / disable trigger to be outputed from the camera to any external device on every depth frame */", "    RS2_OPTION_MOTION_MODULE_TEMPERATURE                  , /**< Current Motion-Module Temperature */", "    RS2_OPTION_DEPTH_UNITS                                , /**< Number of meters represented by a single depth unit */", "    RS2_OPTION_ENABLE_MOTION_CORRECTION                   , /**< Enable/Disable automatic correction of the motion data */", "    RS2_OPTION_AUTO_EXPOSURE_PRIORITY                     , /**< Allows sensor to dynamically ajust the frame rate depending on lighting conditions */", "    RS2_OPTION_COUNT                                      , /**< Number of enumeration values. Not a valid input: intended to be used in for-loops. */"] ("RS Option")
        n38 = event-data() -> ("NewVal"=w105:bool)  [unwired: 1 in, 5 out]
        n39 = Boolean To (0,1)(Boolean=w105) -> (0, 1=w104:i16)
        n40 = call "rs3 set device option.vi"("value"=w104, "RS Option"=w106, "Sensor in"=w107) -> ()  [unwired: 6 in, 3 out]
      }
      event "Autoexposure": Value Change {
        w110 = u16 10 items=["    RS2_OPTION_BACKLIGHT_COMPENSATION                     , /**< Enable / disable color backlight compensation*/", "    RS2_OPTION_BRIGHTNESS                                 , /**< Color image brightness*/", "    RS2_OPTION_CONTRAST                                   , /**< Color image contrast*/", "    RS2_OPTION_EXPOSURE                                   , /**< Controls exposure time of color camera. Setting any value will disable auto exposure*/", "    RS2_OPTION_GAIN                                       , /**< Color image gain*/", "    RS2_OPTION_GAMMA                                      , /**< Color image gamma setting*/", "    RS2_OPTION_HUE                                        , /**< Color image hue*/", "    RS2_OPTION_SATURATION                                 , /**< Color image saturation setting*/", "    RS2_OPTION_SHARPNESS                                  , /**< Color image sharpness setting*/", "    RS2_OPTION_WHITE_BALANCE                              , /**< Controls white balance of color image. Setting any value will disable auto white balance*/", "    RS2_OPTION_ENABLE_AUTO_EXPOSURE                       , /**< Enable / disable color image auto-exposure*/", "    RS2_OPTION_ENABLE_AUTO_WHITE_BALANCE                  , /**< Enable / disable color image auto-white-balance*/", "    RS2_OPTION_VISUAL_PRESET                              , /**< Provide access to several recommend sets of option presets for the depth camera */", "    RS2_OPTION_LASER_POWER                                , /**< Power of the F200 / SR300 projector, with 0 meaning projector off*/", "    RS2_OPTION_ACCURACY                                   , /**< Set the number of patterns projected per frame. The higher the accuracy value the more patterns projected. Increasing the number of patterns help to achieve better accuracy. Note that this c", "    RS2_OPTION_MOTION_RANGE                               , /**< Motion vs. Range trade-off, with lower values allowing for better motion sensitivity and higher values allowing for better depth range*/", "    RS2_OPTION_FILTER_OPTION                              , /**< Set the filter to apply to each depth frame. Each one of the filter is optimized per the application requirements*/", "    RS2_OPTION_CONFIDENCE_THRESHOLD                       , /**< The confidence level threshold used by the Depth algorithm pipe to set whether a pixel will get a valid range or will be marked with invalid range*/", "    RS2_OPTION_EMITTER_ENABLED                            , /**< Laser Emitter enabled */", "    RS2_OPTION_FRAMES_QUEUE_SIZE                          , /**< Number of frames the user is allowed to keep per stream. Trying to hold-on to more frames will cause frame-drops.*/", "    RS2_OPTION_TOTAL_FRAME_DROPS                          , /**< Total number of detected frame drops from all streams */", "    RS2_OPTION_AUTO_EXPOSURE_MODE                         , /**< Auto-Exposure modes: Static, Anti-Flicker and Hybrid */", "    RS2_OPTION_POWER_LINE_FREQUENCY                       , /**< Power Line Frequency control for anti-flickering Off/50Hz/60Hz/Auto */", "    RS2_OPTION_ASIC_TEMPERATURE                           , /**< Current Asic Temperature */", "    RS2_OPTION_ERROR_POLLING_ENABLED                      , /**< disable error handling */", "    RS2_OPTION_PROJECTOR_TEMPERATURE                      , /**< Current Projector Temperature */", "    RS2_OPTION_OUTPUT_TRIGGER_ENABLED                     , /**< Enable / disable trigger to be outputed from the camera to any external device on every depth frame */", "    RS2_OPTION_MOTION_MODULE_TEMPERATURE                  , /**< Current Motion-Module Temperature */", "    RS2_OPTION_DEPTH_UNITS                                , /**< Number of meters represented by a single depth unit */", "    RS2_OPTION_ENABLE_MOTION_CORRECTION                   , /**< Enable/Disable automatic correction of the motion data */", "    RS2_OPTION_AUTO_EXPOSURE_PRIORITY                     , /**< Allows sensor to dynamically ajust the frame rate depending on lighting conditions */", "    RS2_OPTION_COUNT                                      , /**< Number of enumeration values. Not a valid input: intended to be used in for-loops. */"] ("RS Option")
        n41 = event-data() -> ("NewVal"=w109:bool)  [unwired: 1 in, 5 out]
        n42 = Boolean To (0,1)(Boolean=w109) -> (0, 1=w108:i16)
        n43 = call "rs3 set device option.vi"("value"=w108, "RS Option"=w110, "Sensor in"=w111) -> ()  [unwired: 6 in, 3 out]
      }
    }
    n44 = local read "stop"() -> (w78:bool)
  }
  n45 = while {
    tunnel: w54 -> [w168]
    tunnel: w7 -> [w137]
    tunnel: [w139] -> w3
    shift-right: [w135] -> _
    shift-left: sgl[][] [] ("2D Array Output") -> [w159]
    shift-right: [w122] -> _
    shift-left: u8[] [] ("Output Array") -> [w157]
    tunnel: w31 -> [w155]
    tunnel: w30 -> [w154]
    tunnel: w10 -> [w113]
    tunnel: w11 -> [w112]
    shift-right: ["Filter settings"] -> _
    shift-left: T9 {"Decimation Scale (1-10)"=0, "Spatial Alpha\n(0-1)"=0.0, "Spatial Delta \n(1/32 disp)"=0, "Temporal Alpha\n(0-1)"=0.0, "Temporal Delta\n(1/32 disp)"=0, "Persistence (0= none, 8=max)"=0, "spatial holefill radius\n(0 disable, 6 max) "=0, "spatial iteration\n(2=default)"=0} ("Filter settings") -> [w138]
    shift-right: [w142] -> _
    shift-left: T3 {"width"=0, "height"=0, "ppx"=0.0, "ppy"=0.0, "fx"=0.0, "fy"=0.0, "model"=0, "coeffs[0]"=0.0, "coeffs[1]"=0.0, "coeffs[2]"=0.0, "coeffs[3]"=0.0, "coeffs[4]"=0.0} ("intrin post-process out") -> [w147]
    shift-right: ["PostProcess"] -> _
    shift-left: w6 -> [w128]
    shift-right: [w126] -> _
    shift-left: w6 -> [w125]
    tunnel: [w113] -> w4
    tunnel: [w112] -> w1
    i -> [w152]
    stop <- "stop" stop-if-true
    w151 = TRUE ("Transpose")
    # "5B. Post-Process the images \n - Edge preserving Down-sample: it will speed up rendering (try scale=3)\n - Edge preserving edge filter: Will smooth noisy depth\n - Temporal filter: Will average multiple frames using exponential moving average\n - Hole filling: use this carefully, as it is filling in from neighbors\n\nNote: it is always BEST to operate the depth sensor natively at high resolution to \nget the best DEPTH resolution: \nFor D415 you should use 1280x720, and for D435 you should use 848x480\nHowever, it makes sense to down-sample afterward, as this will reduce the X,Y resolution, \nbut wont impact the depth resolution."
    # "8. Release Frames"
    # "7.  Display Frames, but for efficiency only update visible graphs"
    # "6. Interpret frames"
    # "5. Capture Frames"
    n46 = Not Equal?(x=w138, y="Filter settings") -> (x != y?=w150:T16)
    n47 = Cluster To Array(cluster=w150) -> (array=w149:bool[])
    n48 = Or Array Elements(Boolean array=w149) -> (logical OR=w116:bool)
    n49 = case shown="True" w116 {
      tunnel: w113 -> [_ w193]
      tunnel: w137 -> [w189 w192]
      tunnel: [w189 w191] -> w136
      tunnel: "Filter settings" -> [_ w190]
      frame False {
      }
      frame True {
        # "Update Post-Processing\nFilter settings if they change"
        n50 = call "rs3 set filter options.vi"("error in (no error)"=w192, "Processing Blocks"=w193, "Filter settings"=w190) -> ("error out"=w191:errorcluster)  [unwired: 8 in]
      }
    }
    n51 = call "rs3 capture single with post process.vi"("frame queue in"=w168, "Processing Blocks"=w113, "Processing Queues"=w112, "error in (no error)"=w136, "PostProcess"="PostProcess", "Post-processing"="Post-processing") -> ("Capture Error"=→"Capture2 error":string, "Processing times"=w119:T6, "height"=w143:i32, "Processed frame out"=w120:u64, "error out"=w169:errorcluster, "width"=w144:i32, "Stream type"=w160:T17, "intrin post-process out"=w148:T3)  [unwired: 8 in, 6 out]
    n52 = call "rs3 capture single with post process.vi"("frame queue in"=w168, "Processing Blocks"=w113, "Processing Queues"=w112, "error in (no error)"=w169, "PostProcess"="PostProcess", "Post-processing"="Post-processing") -> ("Capture Error"=→"Capture1 Error":string, "Processing times"=w118:T6, "height"=w161:i32, "Processed frame out"=w121:u64, "width"=w162:i32, "Stream type"=w164:T17, "intrin post-process out"=w146:T3)  [unwired: 8 in, 7 out]
    n53 = call "rs3 get frame data2.vi"("frame in"=w120) -> ("error out"=w172:errorcluster, "image pointer out"=w173:u64)  [unwired: 7 in, 2 out]
    n54 = Add(x=w118, y=w119) -> (x+y=→"Processing times":T6)
    n55 = call "rs3 get frame data2.vi"("error in (no error)"=w172, "frame in"=w121) -> ("error out"=w171:errorcluster, "image pointer out"=w163:u64)  [unwired: 6 in, 2 out]
    n56 = case shown="\"Depth\"" w160 {
      tunnel: [w293 w300 w311 w320] -> w165
      tunnel: w173 -> [_ w298 w312 w321]
      tunnel: w144 -> [_ w294 w304 w313]
      tunnel: w143 -> [_ w295 w305 w314]
      tunnel: w171 -> [w293 w301 w310 w319]
      tunnel: [w292 w302 w308 w317] -> w158
      tunnel: w159 -> [w292 _ w308 w317]
      tunnel: w157 -> [w291 w299 _ _]
      tunnel: [w291 w299 w309 w318] -> w156
      tunnel: w151 -> [_ w297 _ _]
      tunnel: w148 -> [_ w296 _ _]
      tunnel: [w290 w296 w306 w315] -> w145
      tunnel: w147 -> [w290 _ w306 w315]
      frame "Color (ext.)", Default {
      }
      frame "Depth" {
        w303 = u16 0 items=["Y16", "Y8"] ("Image format")
        # "Depth"
        n57 = call "rs3_MemCopyUINT16_3.vi"("Image format"=w303, "Transpose"=w297, "error in (no error)"=w301, "Depth Y"=w295, "Depth X"=w294, "Zimage pointer"=w298) -> ("error out"=w300:errorcluster, "2D Array Output"=w302:sgl[][])  [unwired: 2 in, 2 out]
        "Depth height" <- w295
        "Depth width" <- w294
      }
      frame "Color (left) " {
        w307 = enum16{"Monochrome", "RGB internal (RGB)"}."RGB internal (RGB)" ("Color format")
        # "Color"
        n58 = call "rs3_MemCopyRGB_IR2.vi"("Zimage pointer"=w312, "RGB  X, width"=w304, "RGB Y, height"=w305, "Color format"=w307, "error in (no error)"=w310) -> ("Output Array"=w309:u8[], "error out"=w311:errorcluster)  [unwired: 8 in, 1 out]
        n59 = local write "Color format"(w307) -> ()
        "Color Width" <- w304
        "Color Height" <- w305
      }
      frame "IR Left" {
        w316 = enum16{"Monochrome", "RGB internal (RGB)"}."Monochrome" ("Color format")
        # "Mono"
        n60 = local write "Color Width"(w313) -> ()
        n61 = call "rs3_MemCopyRGB_IR2.vi"("Zimage pointer"=w321, "RGB  X, width"=w313, "RGB Y, height"=w314, "Color format"=w316, "error in (no error)"=w319) -> ("Output Array"=w318:u8[], "error out"=w320:errorcluster)  [unwired: 8 in, 1 out]
        n62 = local write "Color format"(w316) -> ()
        n63 = local write "Color Height"(w314) -> ()
      }
    }
    n64 = case shown="\"Color (ext.)\", Default" w164 {
      tunnel: [w261 w268 w280 w289] -> w140
      tunnel: w163 -> [_ w263 w279 w288]
      tunnel: w162 -> [_ w262 w274 w283]
      tunnel: w161 -> [_ w264 w273 w282]
      tunnel: w165 -> [w261 w269 w272 w281]
      tunnel: w158 -> [w260 _ w277 w286]
      tunnel: [w260 w270 w277 w286] -> w135
      tunnel: [w259 w271 w278 w287] -> w122
      tunnel: w156 -> [w259 w271 _ _]
      tunnel: w151 -> [_ w266 _ _]
      tunnel: w146 -> [_ w265 _ _]
      tunnel: w145 -> [w258 _ w275 w284]
      tunnel: [w258 w265 w275 w284] -> w142
      frame "Color (ext.)", Default {
      }
      frame "Depth" {
        w267 = u16 0 items=["Y16", "Y8"] ("Image format")
        # "Depth"
        n65 = local write "Depth height"(w264) -> ()
        n66 = call "rs3_MemCopyUINT16_3.vi"("Image format"=w267, "Transpose"=w266, "error in (no error)"=w269, "Depth Y"=w264, "Depth X"=w262, "Zimage pointer"=w263) -> ("error out"=w268:errorcluster, "2D Array Output"=w270:sgl[][])  [unwired: 2 in, 2 out]
        n67 = local write "Depth width"(w262) -> ()
      }
      frame "Color (left) " {
        w276 = enum16{"Monochrome", "RGB internal (RGB)"}."RGB internal (RGB)" ("Color format")
        # "Color"
        n68 = local write "Color Width"(w274) -> ()
        n69 = call "rs3_MemCopyRGB_IR2.vi"("Zimage pointer"=w279, "RGB  X, width"=w274, "RGB Y, height"=w273, "Color format"=w276, "error in (no error)"=w272) -> ("Output Array"=w278:u8[], "error out"=w280:errorcluster)  [unwired: 8 in, 1 out]
        n70 = local write "Color Height"(w273) -> ()
        n71 = local write "Color format"(w276) -> ()
      }
      frame "IR Left" {
        w285 = enum16{"Monochrome", "RGB internal (RGB)"}."Monochrome" ("Color format")
        # "Mono"
        n72 = local write "Color Width"(w283) -> ()
        n73 = call "rs3_MemCopyRGB_IR2.vi"("Zimage pointer"=w288, "RGB  X, width"=w283, "RGB Y, height"=w282, "Color format"=w285, "error in (no error)"=w281) -> ("Output Array"=w287:u8[], "error out"=w289:errorcluster)  [unwired: 8 in, 1 out]
        n74 = local write "Color Height"(w282) -> ()
        n75 = local write "Color format"(w285) -> ()
      }
    }
    "Processed intrin out" <- w142
    n76 = Unbundle By Name("Post-processing") -> ("Subsample"=w126:bool)
    n77 = First Call?() -> (First Call?: T/F=w115:bool)
    n78 = Not Equal?(x=w128, y="PostProcess") -> (x != y?=w123:bool)
    n79 = Not Equal?(x=w125, y=w126) -> (x != y?=w124:bool)
    n80 = Compound Arithmetic op=OR(w116, w123, w124, w115) -> (w114:bool)
    n81 = And(x=w126, y="PostProcess") -> (x .and. y?=w133:bool)
    n82 = case shown="False" w133 {
      tunnel: w122 -> [w179 w188]
      tunnel: [w179 w187] -> w132
      tunnel: "Filter settings" -> [_ w186]
      tunnel: [w178 w182] -> w129
      tunnel: [w177 w181] -> w131
      frame False {
        n83 = local read "Color Height"() -> (w178:i32)
        n84 = local read "Color Width"() -> (w177:i32)
      }
      frame True {
        # "subsample color image to match depth x,y"
        n85 = local read "Color Height"() -> (w184:i32)
        n86 = local read "Color format"() -> (w180:enum16{"Monochrome", "RGB internal (RGB)"})
        n87 = local read "Color Width"() -> (w183:i32)
        n88 = Unbundle By Name(w186) -> ("Decimation Scale (1-10)"=w185:u8)
        n89 = call "rs3_decimate_color.vi"("Decimate"=w185, "Input X"=w183, "Input Y"=w184, "Color format"=w180, "input image"=w188) -> ("NewX"=w181:i32, "NewY"=w182:i32, "decimated color"=w187:u8[])  [unwired: 4 in]
      }
    }
    n90 = case shown="True" w114 {
      tunnel: w129 -> [_ w174]
      frame False {
      }
      frame True {
        # "Autoscale the Color image\nbut only if values change"
        n91 = property on="RGB image" class="Pict"() -> ("Height"=w175:u32)  [unwired: 2 in, 2 out]
        n92 = Divide(x=w175, y=w174) -> (x/y=w176:dbl)
        n93 = property on="RGB image" class="Pict"("ZoomFactor"=w176) -> ()  [unwired: 2 in, 2 out]
      }
    }
    n94 = case shown="\"PointCloud\"" "Display tab" {
      tunnel: w132 -> [_ w199 w222 _]
      tunnel: w135 -> [_ w194 w206 _]
      tunnel: w155 -> [_ _ w214 _]
      tunnel: w154 -> [_ _ w211 _]
      tunnel: w142 -> [_ _ w204 _]
      tunnel: w129 -> [_ w197 w203 _]
      tunnel: w131 -> [_ w196 w202 _]
      frame "Initialize", Default {
      }
      frame "Color + Depth" {
        (unwired) sgl[][] []  # Blank depthmap
        (unwired) picture bytes[33]  # Blank picture
        n95 = local read "Color format"() -> (w198:enum16{"Monochrome", "RGB internal (RGB)"})
        n96 = call "rs3_RGB_to_Picture5.vi"("RGB array"=w199, "Color format"=w198, "RGB  X, width"=w196, "RGB Y, height"=w197, "AWB"=FALSE, "White Balance"=FALSE) -> ("new picture"=→"RGB image":picture)  [unwired: 8 in, 1 out]
        "Depth map" <- w194
      }
      frame "PointCloud" {
        # "Create x,y,z for PointCloud 3D Picture"
        n97 = Transpose 2D Array(2D array=w206) -> (transposed array=w205:sgl[][])
        n98 = for {
          tunnel: w205 -> [w239] mode=indexing
          tunnel: [w238] -> w217 mode=concatenating
          tunnel: w204 -> [w236]
          i -> [w237]
          n99 = for {
            tunnel: w239 -> [w257] mode=indexing
            tunnel: w237 -> [w256]
            tunnel: [w255] -> w238 mode=indexing
            tunnel: w236 -> [w244]
            i -> [w254]
            n100 = Unbundle By Name(w244) -> ("ppx"=w242:sgl, "ppy"=w243:sgl, "fx"=w240:sgl, "fy"=w241:sgl)
            n101 = To Double Precision Float(number=w256) -> (double precision float=w248:dbl)
            n102 = To Double Precision Float(number=w254) -> (double precision float=w250:dbl)
            n103 = Subtract(x=w250, y=w242) -> (x-y=w249:dbl)
            n104 = Subtract(x=w248, y=w243) -> (x-y=w247:dbl)
            n105 = To Double Precision Float(number=w257) -> (double precision float=w246:dbl)
            n106 = Multiply(x=w246, y=w249) -> (x*y=w253:dbl)
            n107 = Multiply(x=w246, y=w247) -> (x*y=w251:dbl)
            n108 = Divide(x=w253, y=w240) -> (x/y=w252:dbl)
            n109 = Divide(x=w251, y=w241) -> (x/y=w245:dbl)
            n110 = Bundle(w252, w245, w246) -> (w255:cluster{dbl, dbl, dbl})  [unwired: 1 in]
          }
        }
        n111 = case shown="False" "Texture" {
          tunnel: w222 -> [_ w235]
          tunnel: [T14[] [{"Red"=1.0, "Green"=1.0, "Blue"=1.0, "Alpha"=0.0}] ("Color Array") w233] -> w216
          tunnel: "Color format" -> [_ w232]
          tunnel: w202 -> [w224 w231]
          tunnel: w203 -> [w225 w230]
          tunnel: [w223 w229] -> w212
          tunnel: [T15."Overall" ("Color Binding Mode") T15."Per Vertex" ("Color Binding Mode")] -> w208
          frame False {
            n112 = Multiply(x=w225, y=w224) -> (x*y=w223:i32)
          }
          frame True {
            # "Convert color for 3D Picture format"
            n113 = call "rs3_ExtractColor5.vi"("Manual \nWhite Balance"=FALSE ("White Balance"), "24bit Color Array"=w235, "Color format"=w232, "Depth Y"=w230, "RGB  X"=w231, "RGB Y"=w230, "Depth X"=w231) -> ("Norm Mesh Color"=w233:T18)  [unwired: 8 in]
            n114 = Multiply(x=w230, y=w231) -> (x*y=w229:i32)
          }
        }
        n115 = call <vilib>:"Create Mesh.vi"() -> ("New Mesh Refnum"=w219:refnum<vi>)  [unwired: 10 in, 1 out]
        n116 = Array Subset(array=w211, index=0, length=w212) -> (w210:i32[])
        n117 = invoke class="SceneMesh" method="SetMeshParms"(reference=w219, "DrawMode"=T13."Points" ("Draw Mode"), "VertArray"=w217, "Indices"=w210, "ColorMode"=w208, "ColorArray"=w216) -> (reference out=w220:refnum<vi>, error out=w221:errorcluster)  [unwired: 5 in, 9 out]
        n118 = invoke class="SceneObject" method="Set Drawable"(reference=w214, error in=w221, "Drawable"=w220) -> (reference out=→"3D Picture":refnum<vi>)  [unwired: 1 in, 3 out]
      }
      frame "Errors" {
      }
    }
    n119 = call "rs3 release frame.vi"("error in (no error)"=w140, "Frame"=w121) -> ("error out"=w141:errorcluster)  [unwired: 8 in, 1 out]
    n120 = call "rs3 release frame.vi"("error in (no error)"=w141, "Frame"=w120) -> ("error out"=w139:errorcluster)  [unwired: 8 in, 1 out]
    "iteration" <- w152
  }
  n121 = flat-sequence {
    tunnel: [w326] -> w31
    tunnel: [w322] -> w30
    frame #0 {
      # "Cleate Point-Cloud Object"
      n122 = local read "height, Y"() -> (w323:i32)
      n123 = local read "width, X"() -> (w324:i32)
      n124 = call <vilib>:"New Light.vi"("At Infinity"=TRUE) -> ("New Light Refnum"=w334:refnum<vi>)  [unwired: 2 in, 8 out]
      n125 = property class="SceneLight"(reference=w334, "Direction"=cluster{"X":sgl, "Y":sgl, "Z":sgl} {"X"=0.0, "Y"=0.0, "Z"=10000.0}, "Diffuse Color"=T20 {"Alpha"=1.0, "Blue"=1.0, "Green"=1.0, "Red"=1.0}, "atInfinity"=TRUE ("At Infinity"), "Light Number"=0, "Position"=T19 {"X"=10000.0, "Y"=0.0, "Z"=10000.0}, "Specular Color"=T14 {"Red"=1.0, "Green"=0.0, "Blue"=0.0, "Alpha"=0.0}) -> (reference out=w331:refnum<vi>)  [unwired: 1 in, 1 out]
      n126 = call <vilib>:"Create Object (name).vi"("Name"="PointCloud Object") -> ("Scene:New Object"=w333:refnum<vi>)  [unwired: 9 in, 1 out]
      n127 = Multiply(x=w324, y=w323) -> (x*y=w325:i32)
      n128 = for {
        N: w325 -> [_]
        tunnel: [w338] -> w322 mode=indexing
        i -> [w338]
        # "indices"
      }
      n129 = invoke class="SceneObject" method="Light.Add Light"(reference=w333, "Light"=w331) -> (reference out=w326:refnum<vi>)  [unwired: 2 in, 3 out]
    }
  }
  n130 = call "rs3 end processing.vi"("error in (no error)"=w3, "Processing Queues"=w1, "Processing Blocks"=w4) -> ("error out"=w2:errorcluster)  [unwired: 8 in]
  n131 = call "rs3_close all2.vi"("rscontext"=w50, "queue in"=w54, "error in (no error)"=w2, "device_list"=w51, "Dev in"=w36, "Sensor in"=w19) -> ("Close Error"=→"Close Error":string)  [unwired: 4 in, 1 out]
